vi "Switch Display.vi"(8 "error in":errorcluster, 11 "Boolean":refnum<vi>) -> (0 "error out":errorcluster)   [LabVIEW 2018]
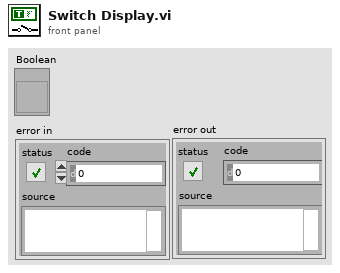
[diagram p1: front panel]
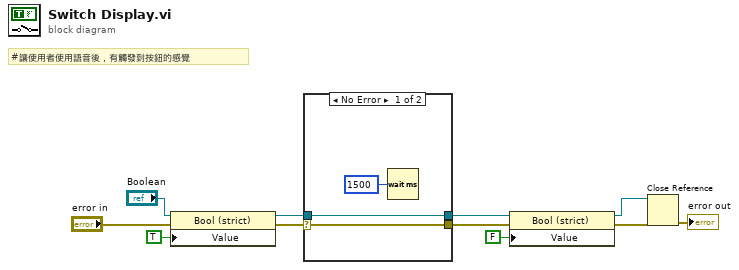
[diagram p0: block diagram]
diagram:
  # "#讓使用者使用語音後，有觸發到按鈕的感覺"
  n1 = property class="Bool (strict)"(reference="Boolean", error in="error in", "Value"=TRUE) -> (reference out=w7:refnum<vi>, error out=w9:errorcluster)
  n2 = case shown="No Error" w9 {
    selector: w9 -> [w14 w16]
    tunnel: [w14 w16] -> w8
    tunnel: w7 -> [w13 w15]
    tunnel: [w13 w15] -> w6
    frame No Error {
      n3 = Wait (ms)(milliseconds to wait=u32 1500) -> ()  [unwired: 1 out]
    }
    frame Error {
    }
  }
  n4 = property class="Bool (strict)"(reference=w6, error in=w8, "Value"=FALSE) -> (reference out=w3:refnum<vi>, error out=w4:errorcluster)
  n5 = Close Reference(reference=w3, error in (no error)=w4) -> (error out=→"error out":errorcluster)
